vi "_PC_Pub_GetCtrlsRef.vi"(3 "error in (no error)":errorcluster, 4 "Ctrls ID":u32[](array[numeric]), 5 "Panel Ref":refnum<vi>) -> (0 "error out":errorcluster, 2 "Ctl Ref Array":refnum<vi>[](array[refnum]))   [LabVIEW 2018]
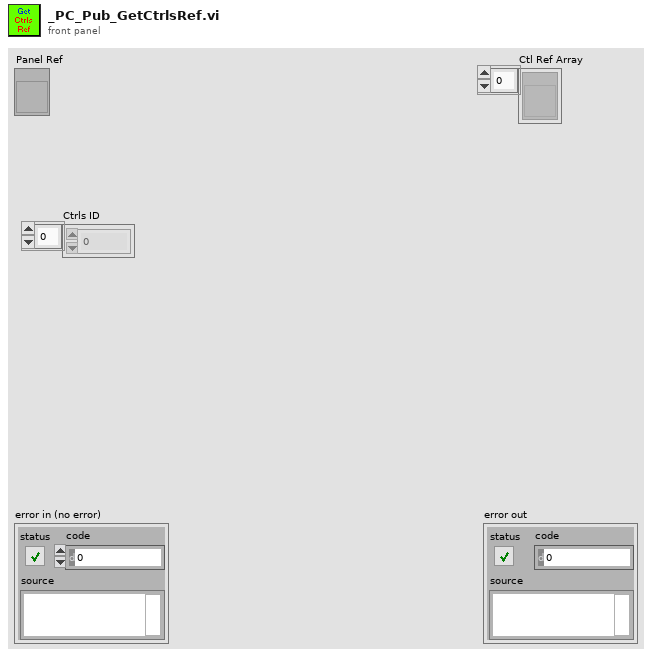
[diagram p1: front panel]
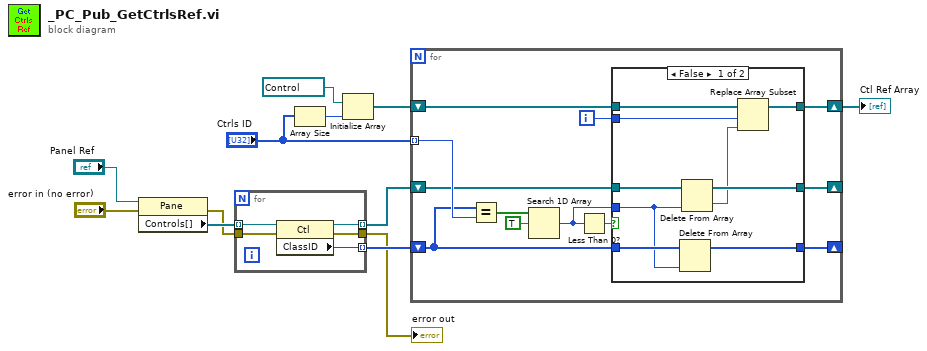
[diagram p0: block diagram]
diagram:
  n1 = property class="Pane"(reference="Panel Ref", error in="error in (no error)") -> (error out=w5:errorcluster, "Controls[]"=w6:refnum<vi>[])  [unwired: 1 out]
  n2 = for {
    tunnel: w6 -> [w17] mode=indexing
    tunnel: w5 -> [w16]
    tunnel: [w15] -> w1
    tunnel: [w14] -> w4 mode=indexing
    tunnel: [w13] -> w3 mode=indexing
    n3 = property class="Ctl"(reference=w17, error in=w16) -> (reference out=w13:refnum<vi>, error out=w15:errorcluster, "ClassID"=w14:u32)
  }
  "error out" <- w1
  n4 = Array Size(array="Ctrls ID") -> (size(s)=w9:i32)
  n5 = Initialize Array(refnum<vi> refnum ("reference out"), w9) -> (w8:refnum<vi>[])
  n6 = for {
    tunnel: "Ctrls ID" -> [w24] mode=indexing
    shift-right: [w25] -> w7
    shift-left: w8 -> [w26]
    shift-right: [w19] -> _
    shift-left: w4 -> [w20]
    shift-right: [w18] -> _
    shift-left: w3 -> [w23]
    i -> [w22]
    n7 = Equal?(x=w20, y=w24) -> (x = y?=w29:bool[])
    n8 = Search 1D Array(1D array=w29, element=TRUE) -> (index of element=w21:i32)  [unwired: 1 in]
    n9 = Less Than 0?(x=w21) -> (x < 0?=w27:bool)
    n10 = case shown="False" w27 {
      tunnel: w26 -> [w38 w41]
      tunnel: w23 -> [w33 w39]
      tunnel: [w37 w41] -> w25
      tunnel: w22 -> [w36 _]
      tunnel: w21 -> [w32 _]
      tunnel: w20 -> [w35 w40]
      tunnel: [w34 w40] -> w19
      tunnel: [w31 w39] -> w18
      frame False {
        n11 = Delete From Array(array=w35, index=w32) -> (array with subset deleted=w34:u32[])  [unwired: 1 in, 1 out]
        n12 = Delete From Array(array=w33, index=w32) -> (deleted portion=w30:refnum<vi>, array with subset deleted=w31:refnum<vi>[])  [unwired: 1 in]
        n13 = Replace Array Subset(array=w38, new element=w30, index=w36) -> (w37:refnum<vi>[])
      }
      frame True {
      }
    }
  }
  "Ctl Ref Array" <- w7
